vi "Error Test Direction.vi"(8 "error in":errorcluster, 10 "direction":string) -> (0 "error out":errorcluster)   [LabVIEW 2020, in "Ballard ARINC 429 Import.lvlib"]
uses:
  Ballard ARINC 429 Import.lvlib
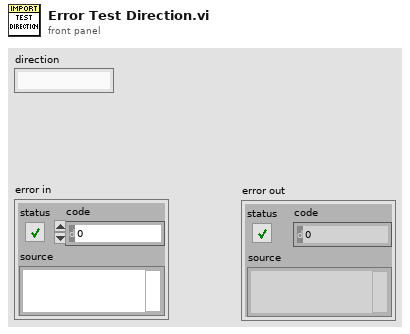
[diagram p1: front panel]
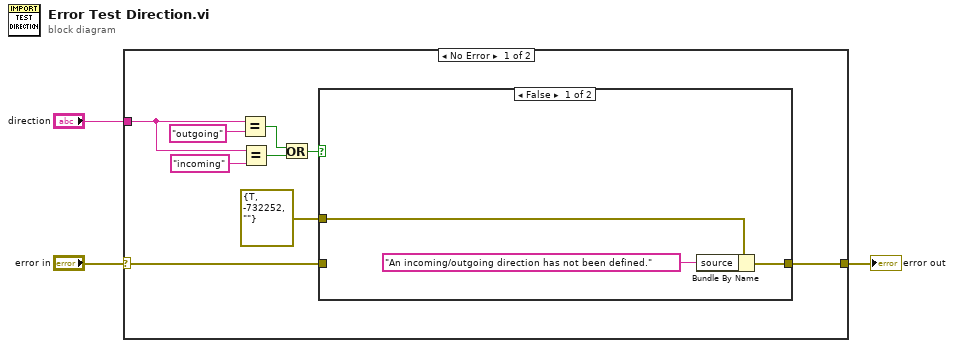
[diagram p0: block diagram]
diagram:
  n1 = case shown="No Error" "error in" {
    selector: "error in" -> [w11 w17]
    tunnel: [w10 w17] -> w2
    tunnel: "direction" -> [w12 _]
    frame No Error {
      n2 = Equal?(x=w12, y="outgoing") -> (x = y?=w8:bool)
      n3 = Equal?(x=w12, y="incoming") -> (x = y?=w7:bool)
      n4 = Or(x=w8, y=w7) -> (x .or. y?=w4:bool)
      n5 = case shown="False" w4 {
        tunnel: errorcluster {"status"=TRUE, "code"=-732252, "source"=""} ("error constant") -> [w15 _]
        tunnel: [w14 w16] -> w10
        tunnel: w11 -> [_ w16]
        frame False {
          n6 = Bundle By Name(cluster=w15, "source"="An incoming/outgoing direction has not been defined.") -> (w14:errorcluster)
        }
        frame True {
        }
      }
    }
    frame Error {
    }
  }
  "error out" <- w2
